vi "Twitter Open.vi"(4 "Access Token Secret (In)":string, 6 "Access Token (In)":string, 8 "error in":errorcluster, 10 "Consumer Secret":string, 11 "Consumer Key":string) -> (0 "error out":errorcluster, 1 "Access Token Secret (Out)":string, 2 "Access Token (Out)":string, 3 "Twitter Handle Out":T1={"OAuth Credentials"={"Consumer Key"="", "Signature Method"=enum."HMAC-SHA1", "Token"="", "Version"="", "Token Secret"="", "Consumer Secret"=""}, "since ID"="", "max ID"="", "Screen Name"=""})   [LabVIEW 2011, in "i3-twitter.lvlib"]
uses:
  i3-twitter.lvlib
  Controls/Twitter Handle.ctl
  i3-oauth/Controls/OAuth Credentials.ctl
  i3-oauth/Controls/Signature Method.ctl
  i3-oauth/i3-oauth.lvlib
panel:
  out "Response Header":string
  out "Response Body":string
  # "Debug Only"
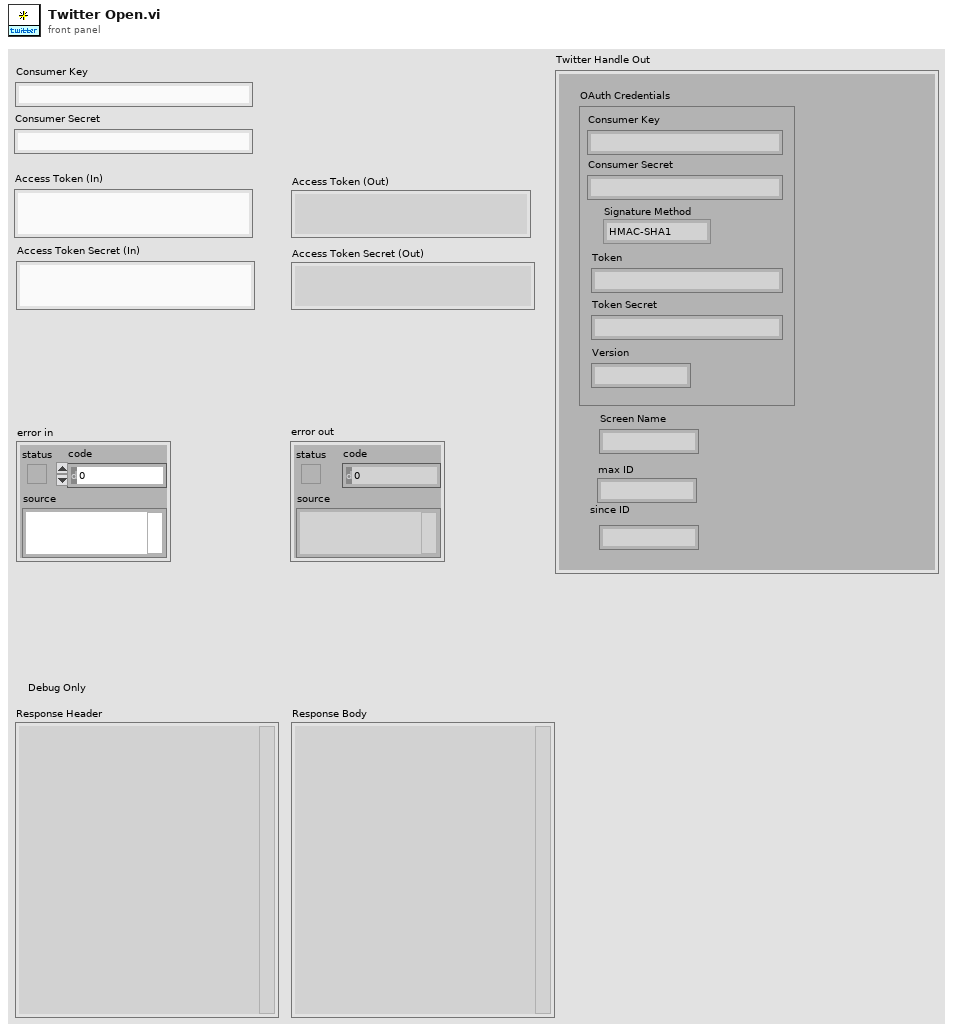
[diagram p1: front panel]
types:
  T1 = typedef "i3-twitter.lvlib/Twitter Handle.ctl" = cluster{"OAuth Credentials":T2, "since ID":string, "max ID":string, "Screen Name":string}
  T2 = typedef "i3-oauth.lvlib/OAuth Credentials.ctl" = cluster{"Consumer Key":string, "Signature Method":T3, "Token":string, "Version":string, "Token Secret":string, "Consumer Secret":string}
  T3 = typedef "i3-oauth.lvlib/Signature Method.ctl" = enum16{"HMAC-MD5", "HMAC-SHA1", "HMAC-SHA224", "HMAC-SHA256", "HMAC-SHA384", "HMAC-SHA512"}
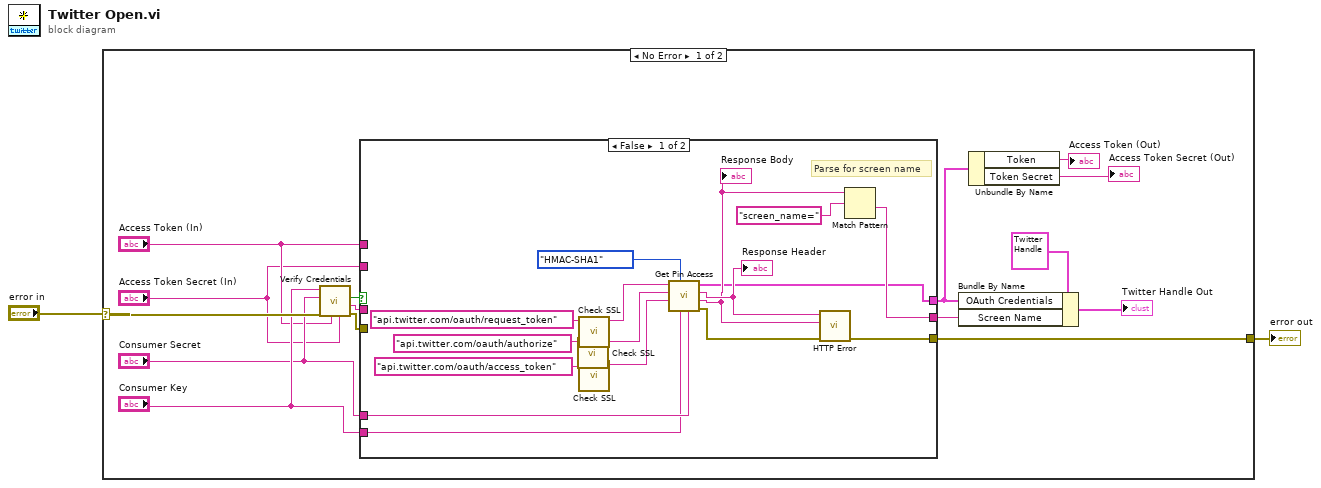
[diagram p0: block diagram]
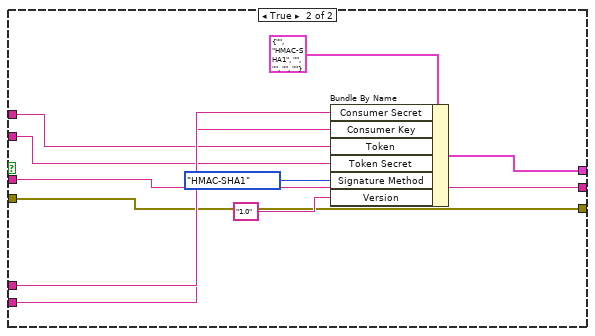
[diagram p2: hidden frame]
diagram:
  n1 = case shown="No Error" "error in" {
    selector: "error in" -> [w7 w44]
    tunnel: [w16 w44] -> w2
    frame No Error {
      n2 = call "Verify Credentials.vi"("Access Token Secret (In)"="Access Token Secret (In)", "Access Token (In)"="Access Token (In)", "error in (no error)"=w7, "Consumer Secret"="Consumer Secret", "Consumer Key"="Consumer Key") -> ("error out"=w13:errorcluster, "Screen Name"=w12:string, "Success?"=w17:bool)  [unwired: 3 in, 1 out]
      n3 = case shown="False" w17 {
        tunnel: "Consumer Secret" -> [w19 w43]
        tunnel: "Consumer Key" -> [w18 w42]
        tunnel: "Access Token (In)" -> [_ w41]
        tunnel: "Access Token Secret (In)" -> [_ w40]
        tunnel: [w21 w37] -> w11
        tunnel: [w31 w35] -> w16
        tunnel: [w33 w34] -> w14
        tunnel: w13 -> [_ w35]
        tunnel: w12 -> [_ w34]
        frame False {
          # "Parse for screen name"
          n4 = call "Check SSL.vi"("Input URL"="api.twitter.com/oauth/authorize" ("Authorize URL")) -> ("Output URL"=w25:string)  [unwired: 8 in]
          n5 = call "Check SSL.vi"("Input URL"="api.twitter.com/oauth/request_token" ("Request URL")) -> ("Output URL"=w28:string)  [unwired: 8 in]
          n6 = call "Check SSL.vi"("Input URL"="api.twitter.com/oauth/access_token" ("Access URL")) -> ("Output URL"=w26:string)  [unwired: 8 in]
          n7 = call "Get Pin Access.vi"("Consumer Secret"=w19, "Consumer Key"=w18, "Signature Method"=Signature_Method."HMAC-SHA1", "Access URL"=w26, "Authorize URL"=w25, "Request URL"=w28) -> ("error out"=w32:errorcluster, "body"=w22:string, "headers"=w23:string, "OAuth Credentials"=w21:T2)  [unwired: 2 in]
          "Response Body" <- w22
          "Response Header" <- w23
          n8 = call "HTTP Error.vi"("error in (no error)"=w32, "Body"=w22, "Header"=w23) -> ("error out"=w31:errorcluster)  [unwired: 6 in, 2 out]
          n9 = Match Pattern(string=w22, regular expression="screen_name=" ("format string")) -> (after substring=w33:string)  [unwired: 1 in, 3 out]
        }
        frame True {
          n10 = Bundle By Name(cluster=T2 {"Consumer Key"="", "Signature Method"=enum."HMAC-SHA1", "Token"="", "Version"="", "Token Secret"="", "Consumer Secret"=""} ("OAuth Credentials"), "Consumer Secret"=w43, "Consumer Key"=w42, "Token"=w41, "Token Secret"=w40, "Signature Method"=Signature_Method."HMAC-SHA1", "Version"="1.0") -> (w37:T2)
        }
      }
      n11 = Bundle By Name(cluster=T1 {"OAuth Credentials"={"Consumer Key"="", "Signature Method"=enum."HMAC-MD5", "Token"="", "Version"="", "Token Secret"="", "Consumer Secret"=""}, "since ID"="", "max ID"="", "Screen Name"=""} ("Twitter Handle"), "OAuth Credentials"=w11, "Screen Name"=w14) -> (→"Twitter Handle Out":T1)
      n12 = Unbundle By Name(w11) -> ("Token"=→"Access Token (Out)":string, "Token Secret"=→"Access Token Secret (Out)":string)
    }
    frame Error {
    }
  }
  "error out" <- w2
